vi "RF Characterization UI.vi"() -> ()   [LabVIEW 2010]
uses:
  <vilib>/Utility/file.llb/Write To Spreadsheet File (DBL).vi
panel:
  in  "Gantry Accel/Decel":dbl=5.0
  in  "Gantry Velocity":dbl=5.0
  in  "Z Range":cluster{"Min":dbl, "Max":dbl, "Increment":dbl}={"Min"=0.0, "Max"=0.0, "Increment"=1.0}
  in  "Y Range":cluster{"Min":dbl, "Max":dbl, "Increment":dbl}={"Min"=-5.0, "Max"=5.0, "Increment"=0.25}
  in  "X Range":cluster{"Min":dbl, "Max":dbl, "Increment":dbl}={"Min"=1.0, "Max"=20.0, "Increment"=0.25}
  in  "MICS Power":u8=31 format="%.0x"
  out "Intensity Graph":dbl[][](graph)
  in  "Z Layer":i32
  out "error out":errorcluster
  in  "Samples":i32=5
  in  "Attenuation (dB)":dbl
  out "Bad Position":bool
  in  "error in (no error)":errorcluster
  in  "stop":bool
  in  "TARGET MICS ID":u32=4358 format="%.0x"
  in  "VISA Resource Name":refnum<visa-resource-name>="COM5"
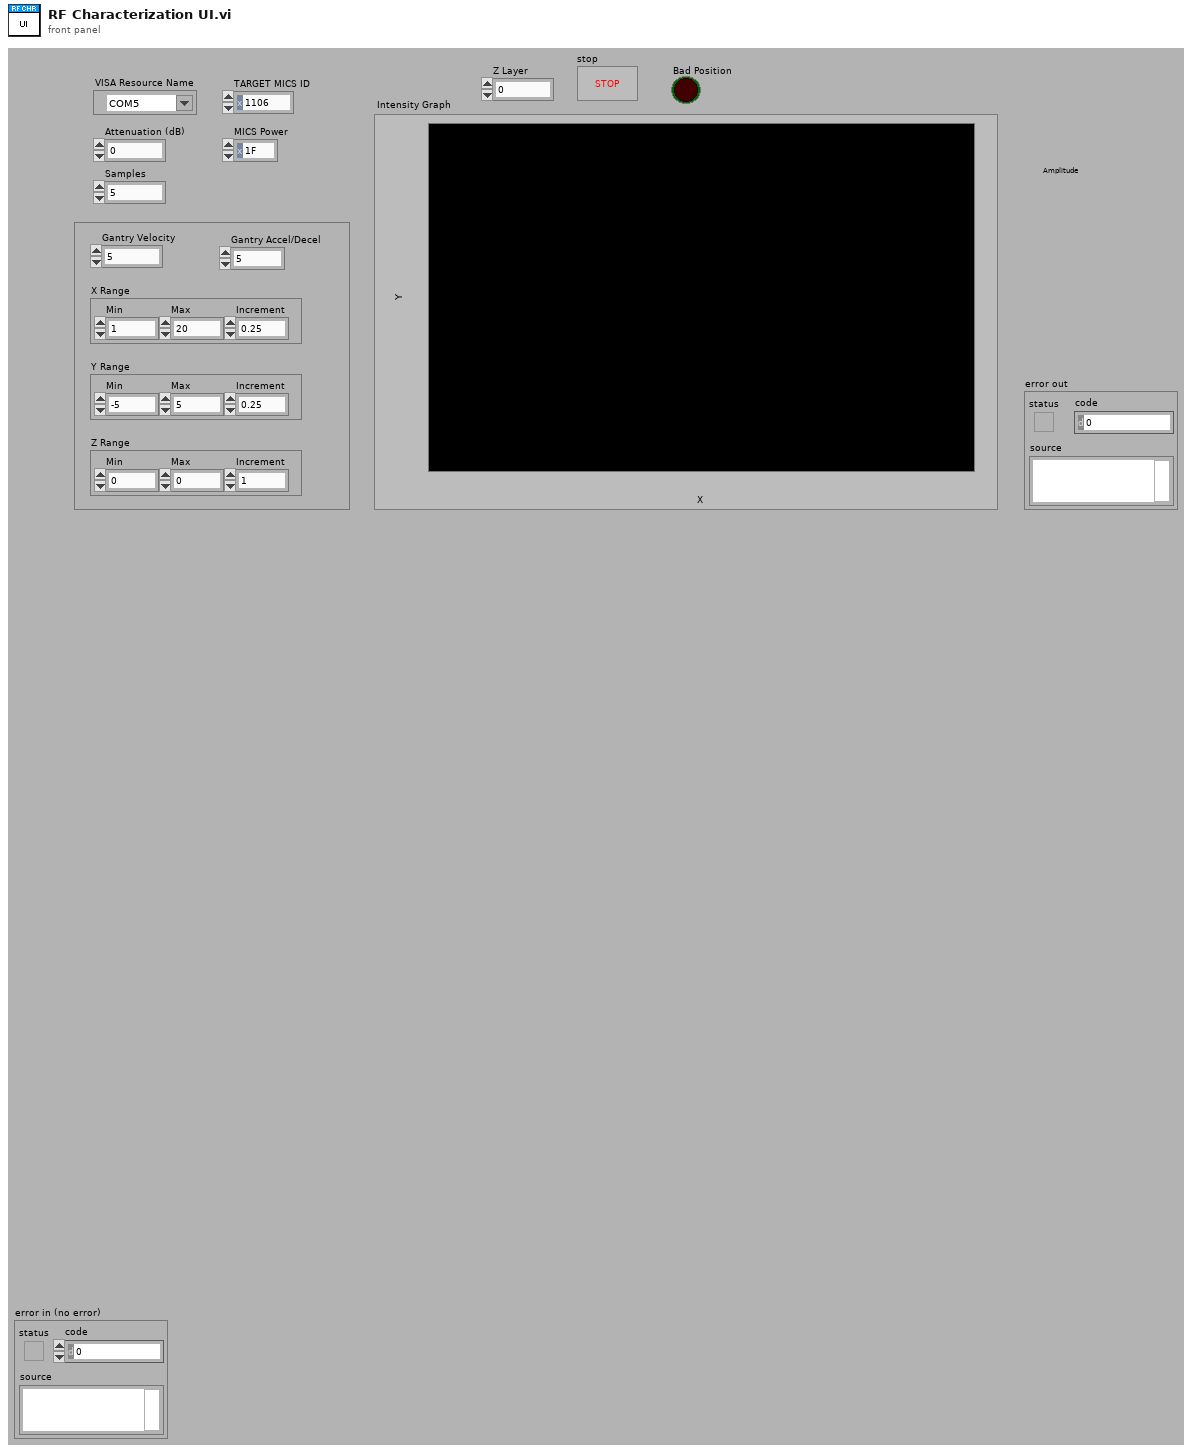
[diagram p1: front panel]
types:
  T1 = typedef "Motion_Gantry Position.ctl" = cluster{"Gantry Accel/Decel":dbl, "Gantry Velocity":dbl, "X-Position":dbl, "Y-Position":dbl, "Z-Position":dbl}
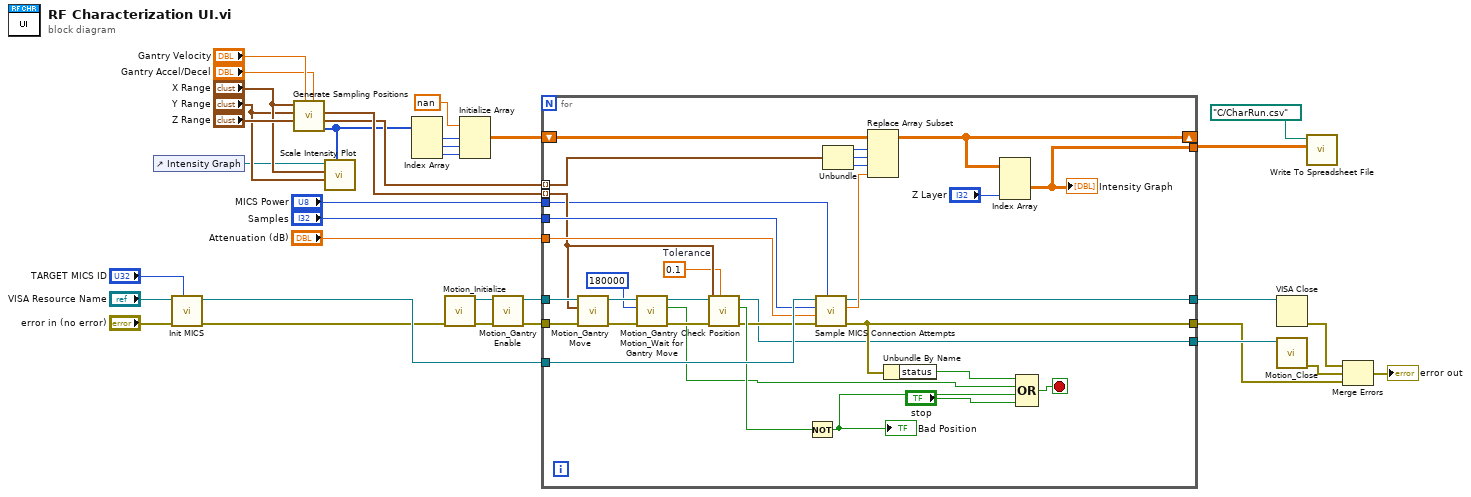
[diagram p0: block diagram]
diagram:
  n1 = control-ref of="Intensity Graph"() -> (w20:refnum<vi>)
  n2 = call "Init MICS.vi"("TARGET MICS ID"="TARGET MICS ID", "error in (no error)"="error in (no error)", "VISA Resource Name"="VISA Resource Name") -> ("error out"=w5:errorcluster, "dup VISA Resource Name"=w6:refnum<visa-resource-name>)  [unwired: 7 in]
  n3 = call "Generate Sampling Positions.vi"("Gantry Accel/Decel"="Gantry Accel/Decel", "Gantry Velocity"="Gantry Velocity", "Z Range"="Z Range", "Y Range"="Y Range", "X Range"="X Range") -> ("Dimensions"=w13:i32[], "Indices"=w28:cluster{i32, i32, i32}[], "Output"=w30:T1[])  [unwired: 4 in]
  n4 = call "Scale Intensity Plot.vi"("Dimensions"=w13, "Y Range"="Y Range", "X Range"="X Range", "IntGraph Refnum"=w20) -> ()  [unwired: 6 in, 2 out]
  n5 = Index Array(array=w13) -> (element #1=w27:i32, element #2=w26:i32, element #3=w25:i32)  [unwired: 3 in]
  n6 = call "Motion_Initialize.vi"("error in (no error)"=w5) -> ("error out"=w1:errorcluster, "connection ID"=w4:refnum<k5>)  [unwired: 9 in]
  n7 = Initialize Array(nan ("element"), w27, w26, w25) -> (w23:dbl[][][])
  n8 = call "Motion_Gantry Enable.vi"("error in (no error)"=w1, "TCP Connection Refnum in"=w4) -> ("error out"=w2:errorcluster, "TCP Connection Refnum (dup)"=w3:refnum<k5>)  [unwired: 8 in]
  n9 = for {
    tunnel: w6 -> [w54]
    tunnel: [w51] -> w34
    tunnel: [w53] -> w15
    tunnel: w3 -> [w65]
    tunnel: [w36] -> w17
    tunnel: w2 -> [w63]
    tunnel: w30 -> [w42] mode=indexing
    tunnel: w28 -> [w61] mode=indexing
    shift-right: [w57] -> _
    shift-left: w23 -> [w62]
    tunnel: [w55] -> w19
    tunnel: "Samples" -> [w49]
    tunnel: "Attenuation (dB)" -> [w47]
    tunnel: "MICS Power" -> [w35]
    stop <- w64 stop-if-true
    w37 = 0.1  # Tolerance
    n10 = call "Motion_Gantry Move.vi"("error in (no error)"=w63, "Gantry Move Data"=w42, "TCP Connection Refnum in"=w65) -> ("error out"=w45:errorcluster, "TCP Connection Refnum (dup)"=w46:refnum<k5>)  [unwired: 7 in]
    n11 = call "Motion_Wait for Gantry Move.vi"("error in (no error)"=w45, "Timeout sec (-1 = No timeout)"=180000 ("Timeout ms (-1 = No timeout)"), "TCP Connection Refnum in"=w46) -> ("error out"=w41:errorcluster, "Timed Out?"=w38:bool, "TCP Connection Refnum (dup)"=w43:refnum<k5>)  [unwired: 5 in, 1 out]
    n12 = call "Motion_Gantry Check Position.vi"("Tolerance (0.1)"=w37, "error in (no error)"=w41, "Gantry Move Data"=w42, "TCP Connection Refnum"=w43) -> ("error out"=w39:errorcluster, "In Position?"=w40:bool, "TCP Connection Refnum (dup)"=w36:refnum<k5>)  [unwired: 5 in]
    n13 = Not(x=w40) -> (.not. x?=w50:bool)
    "Bad Position" <- w50
    n14 = call "Sample MICS Connection Attempts.vi"("MICS Power Setting (0x1F)"=w35, "error in"=w39, "Attenuation dB"=w47, "Samples (1)"=w49, "MICS Resource Name"=w54) -> ("error out"=w53:errorcluster, "Percent Successful"=w52:dbl, "MICS Resource Name out"=w51:refnum<visa-resource-name>)  [unwired: 3 in, 1 out]
    n15 = Unbundle(w61) -> (w60:i32, w59:i32, w58:i32)
    n16 = Replace Array Subset(array=w62, new element=w52, index (dim 0)=w60, index (dim 1)=w59, index (dim 2)=w58) -> (w57:dbl[][][])
    n17 = Unbundle By Name(w53) -> ("status"=w66:bool)
    n18 = Index Array(array=w57, index (dim 2)="Z Layer") -> (element=w55:dbl[][])  [unwired: 2 in]
    "Intensity Graph" <- w55
    n19 = Compound Arithmetic op=OR(w66, w38, w50, "stop") -> (w64:bool)
  }
  n20 = VISA Close(VISA resource name=w34) -> (error out=w29:errorcluster)  [unwired: 1 in]
  n21 = call "Motion_Close.vi"("connection ID"=w17) -> ("error out"=w16:errorcluster)  [unwired: 10 in]
  n22 = call-poly <vilib>:"Write To Spreadsheet File.vi"("2D data"=w19, "file path (dialog if empty)"=path "C:/CharRun.csv") -> ()  [unwired: 6 in, 1 out]
  n23 = Merge Errors(w29, w16, w15) -> (→"error out":errorcluster)
